vi "SD Read String.vi"(8 "error in":errorcluster, 10 "Table Prefix":string="SmartDashboard", 11 "Name":string="String") -> (0 "error out":errorcluster, 2 "Table Prefix out":string, 3 "String":string)   [LabVIEW 2017]
doc: "Return the string data stored in the SmartDashboard entry -- /prefix/name. Return an error if not present or not a string."
uses:
  <vilib>/Rock Robotics/Network Tables/Field Type.ctl
  <vilib>/Rock Robotics/Network Tables/Field Data Manager.vi
  <vilib>/Rock Robotics/Network Tables/Table Manager.vi
  <vilib>/Rock Robotics/Network Tables/Prepare Table Name.vi
  <vilib>/Rock Robotics/Network Tables/Usage Statistics.vi
  <vilib>/Rock Robotics/Network Tables/NT Globals.vi
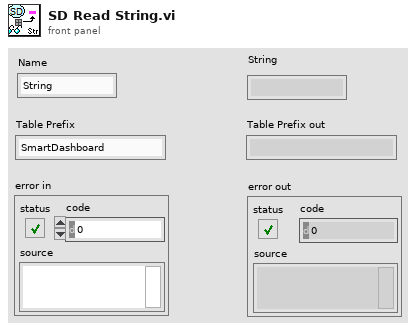
[diagram p1: front panel]
types:
  T1 = typedef "Field Type.ctl" = enum8{"Invalid", "Bool", "Numeric", "String", "Raw", "Boolean Array", "Numeric Array", "String Array", "RPC"}
  T2 = typedef "Field Data.ctl" = cluster{"Dbl":dbl, "String":string, "Type":T1, "Boolean":bool, "Sequence #":T3, "Flags":u8}
  T3 = typedef "Sequence.ctl" = u16
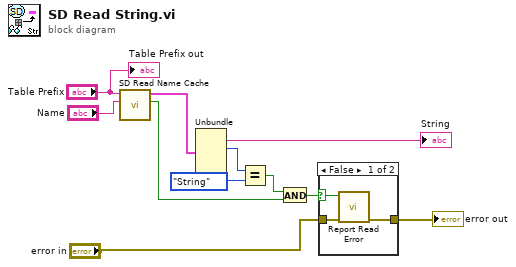
[diagram p0: block diagram]
diagram:
  n1 = call <vilib>:"SD Read Name Cache.vi"("Name"="Name", "Table Prefix"="Table Prefix") -> ("Success"=w11:bool, "Field Value Out"=w10:T2)  [unwired: 8 in]
  n2 = Unbundle(w10) -> ("String"=→"String":string, "Type"=w7:T1)  [unwired: 4 out]
  n3 = Equal?(x=w7, y=Field_Type."String" ("Type")) -> (x = y?=w9:bool)
  n4 = And(x=w9, y=w11) -> (x .and. y?=w6:bool)
  n5 = case shown="False" w6 {
    selector: w6 -> [w12 _]
    tunnel: [w14 w15] -> w2
    tunnel: "error in" -> [w13 w15]
    frame False {
      n6 = call <vilib>:"Report Read Error.vi"("error in (no error)"=w13, "Success"=w12) -> ("error out"=w14:errorcluster)  [unwired: 9 in]
    }
    frame True {
    }
  }
  "error out" <- w2
  "Table Prefix out" <- "Table Prefix"
